vi "Check Job Input Buffer.vi"(5 "First Call?":bool, 6 "error in":errorcluster, 9 "Input Buffer":path) -> (0 "error out":errorcluster, 2 "Jobs":string[](array[string]), 3 "Input Buffer Out":path)   [LabVIEW 2015]
panel:
  out "New Jobs":string[](array[string])
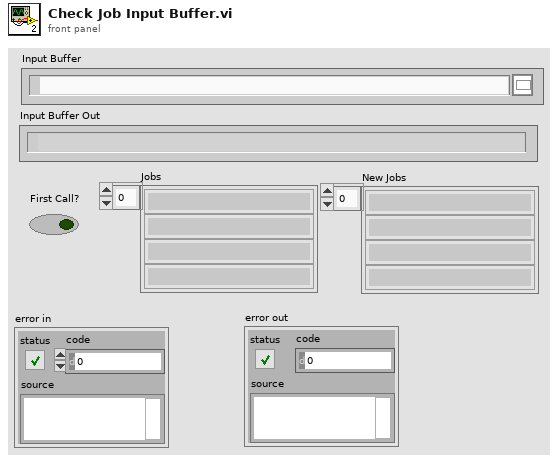
[diagram p1: front panel]
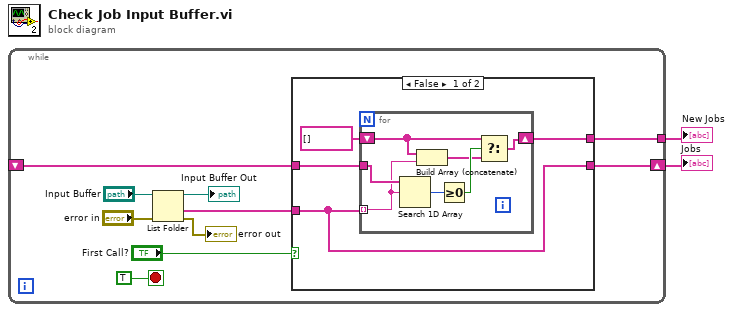
[diagram p0: block diagram]
diagram:
  n1 = while {
    shift-right: [w10] -> w1
    shift-left: _ -> [w9]
    tunnel: [w4] -> w2
    stop <- TRUE stop-if-true
    n2 = List Folder(path="Input Buffer", error in="error in") -> (path out=→"Input Buffer Out":path, folder names=w6:string[], error out=→"error out":errorcluster)  [unwired: 2 in, 1 out]
    n3 = case shown="False" "First Call?" {
      tunnel: [w14 w24] -> w10
      tunnel: w9 -> [w16 _]
      tunnel: w6 -> [w14 w24]
      tunnel: [w15 _] -> w4
      frame False {
        n4 = for {
          tunnel: w16 -> [w23]
          tunnel: w14 -> [w19] mode=indexing
          shift-right: [w20] -> w15
          shift-left: string[] [] -> [w18]
          n5 = Search 1D Array(1D array=w23, element=w19) -> (index of element=w22:i32)  [unwired: 1 in]
          n6 = Build Array (concatenate)(w18, w19) -> (w17:string[])
          n7 = Greater Or Equal To 0?(x=w22) -> (x >= 0?=w21:bool)
          n8 = Select(t=w18, s=w21, f=w17) -> (s? t:f=w20:string[])
        }
      }
      frame True {
      }
    }
  }
  "Jobs" <- w1
  "New Jobs" <- w2
